vi "TBQ_ComputeMinMax.vi"(11 "TimeBasedQueue In":refnum<class "TimeBasedQueue.lvclass">) -> (0 "Minimum":dbl format="%0.2f", 1 "Maximum":dbl format="%0.2f", 3 "TimeBasedQueue Out":refnum<class "TimeBasedQueue.lvclass">)   [LabVIEW 2012, in "TimeBasedQueue.lvclass"]
uses:
  TimeBasedQueue.lvclass
  TimeBasedQueue.lvclass/TimeBasedQueue.ctl
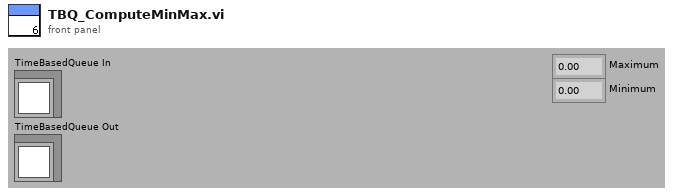
[diagram p1: front panel]
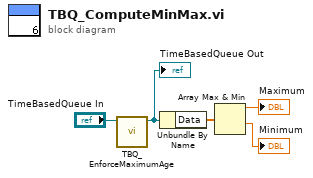
[diagram p0: block diagram]
diagram:
  n1 = call "TBQ_EnforceMaximumAge.vi"("TimeBasedQueue In"="TimeBasedQueue In") -> ("TimeBasedQueue Out"=w4:refnum<class "TimeBasedQueue.lvclass">)  [unwired: 10 in]
  "TimeBasedQueue Out" <- w4
  n2 = Unbundle By Name(w4) -> ("Data"=w3:dbl[])
  n3 = Array Max & Min(array=w3) -> (max value=→"Maximum":dbl, min value=→"Minimum":dbl)  [unwired: 2 out]
